vi "Start.vi"(8 "error in (no error)":errorcluster, 11 "Thermometer DAQmx Base CFG in":refnum<class "Thermometer DAQmx Base CFG.lvclass">) -> (0 "error out":errorcluster, 3 "Thermometer DAQmx Base CFG out":refnum<class "Thermometer DAQmx Base CFG.lvclass">)   [LabVIEW 2023, in "Thermometer DAQmx Base CFG.lvlib" / "Thermometer DAQmx Base CFG.lvclass"]
uses:
  Thermometer DAQmx Base CFG.lvclass
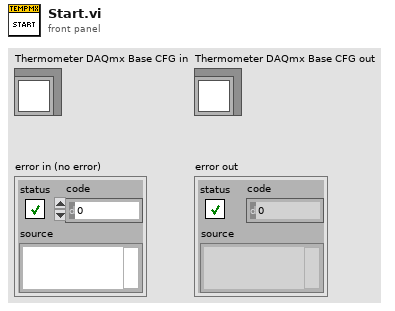
[diagram p1: front panel]
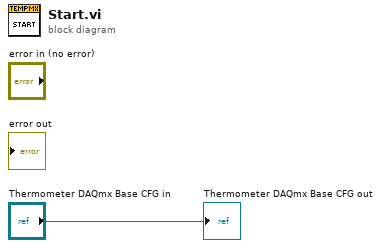
[diagram p0: block diagram]
diagram:
  "Thermometer DAQmx Base CFG out" <- "Thermometer DAQmx Base CFG in"
